vi "Filter Calc.vi"(8 "error in (no error)":errorcluster, 9 "Node Data":T2, 10 "Node Path (parent, child)":string[](array[string]), 11 "Filter in":refnum<class "Filter.lvclass">) -> (0 "error out":errorcluster, 1 "Keep options":T1, 2 "Keep node?":bool, 3 "Filter out":refnum<class "Filter.lvclass">)   [LabVIEW 2020, in "Blue Tree Map OpenSource.lvlib" / "Filter.lvclass"]
uses:
  Filter.lvclass
  Typedefs/Tree Node Data.ctl
  Typedefs/Attribute Map.ctl
  Typedefs/Filter calc option.ctl
  Blue Tree Map OpenSource.lvlib
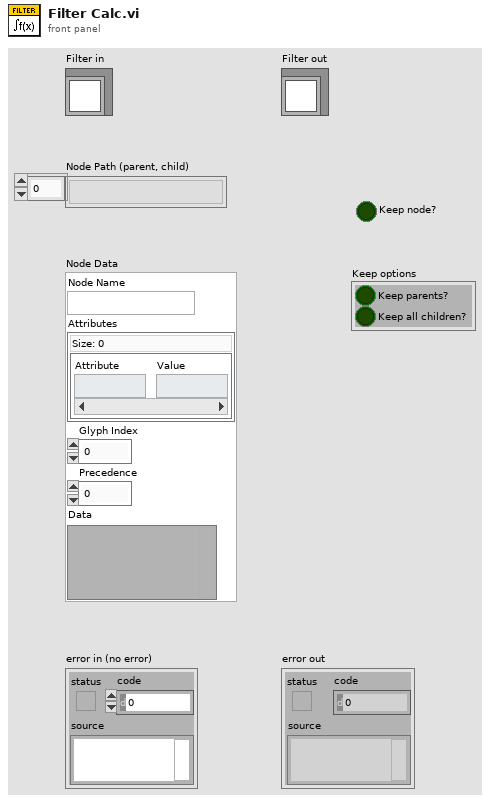
[diagram p1: front panel]
types:
  T1 = typedef "Blue Tree Map OpenSource.lvlib/Filter calc option.ctl" = cluster{"Keep parents?":bool, "Keep all children?":bool}
  T2 = typedef "Blue Tree Map OpenSource.lvlib/Tree Node Data.ctl" = cluster{"Node Name":string, "Attributes":T3, "Glyph Index":i32, "Precedence":i32, "Data":variant}
  T3 = typedef "Blue Tree Map OpenSource.lvlib/Attribute Map.ctl" = map{string, string}
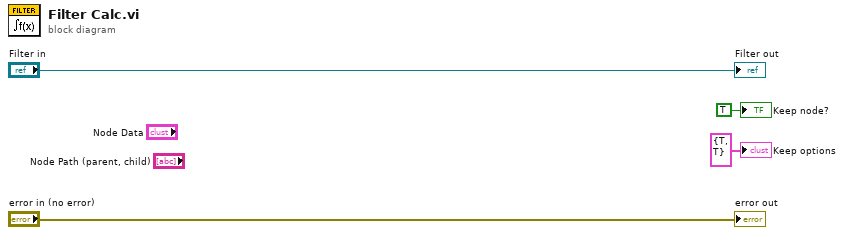
[diagram p0: block diagram]
diagram:
  "error out" <- "error in (no error)"
  "Filter out" <- "Filter in"
  "Keep options" <- T1 {"Keep parents?"=TRUE, "Keep all children?"=TRUE} ("Keep options")
  "Keep node?" <- TRUE ("Keep node?")
